vi "fill_tree.vi"(0 "Tree Refnum":refnum<vi>, 1 "Match String":string, 5 "Command Spec":T1, 7 "Operation":u16(ring) items=["Rebuild", "Add Items"], 9 "Property":string[](array[string]), 11 "Available Commands Pool":refnum<vi>, 12 "Group":string[](array[string]), 13 "Items to Insert":string[](array[string]), 14 "Sorting Method":u16) -> ()   [LabVIEW 2018]
uses:
  command_spec.ctl
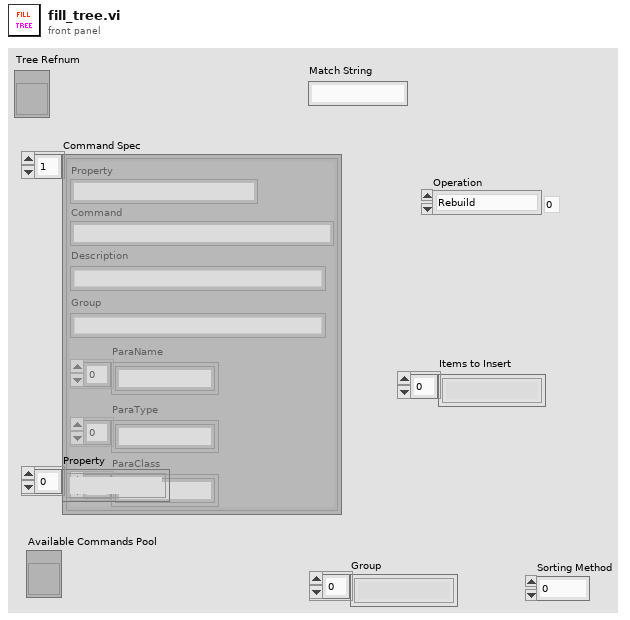
[diagram p1: front panel]
types:
  T1 = typedef "command_spec.ctl" = cluster{"Property":string, "Command":string, "Description":string, "Group":string, "ParaName":string[], "ParaType":string[], "ParaClass":string[]}[]
  T2 = cluster{"Left Cell String":string, "Child Text":string[], "Child Tag":string, "Item Indent":i32, "Child Only?":bool, "Glyph Index":i32}[]
  T3 = cluster{"Left Cell String":string, "Child Text":string[], "Child Tag":string, "Item Indent":i32, "Child Only?":bool, "Glyph Index":i32}
  T4 = cluster{"Property":string, "Command":string, "Description":string, "Group":string, "ParaName":string[], "ParaType":string[], "ParaClass":string[]}
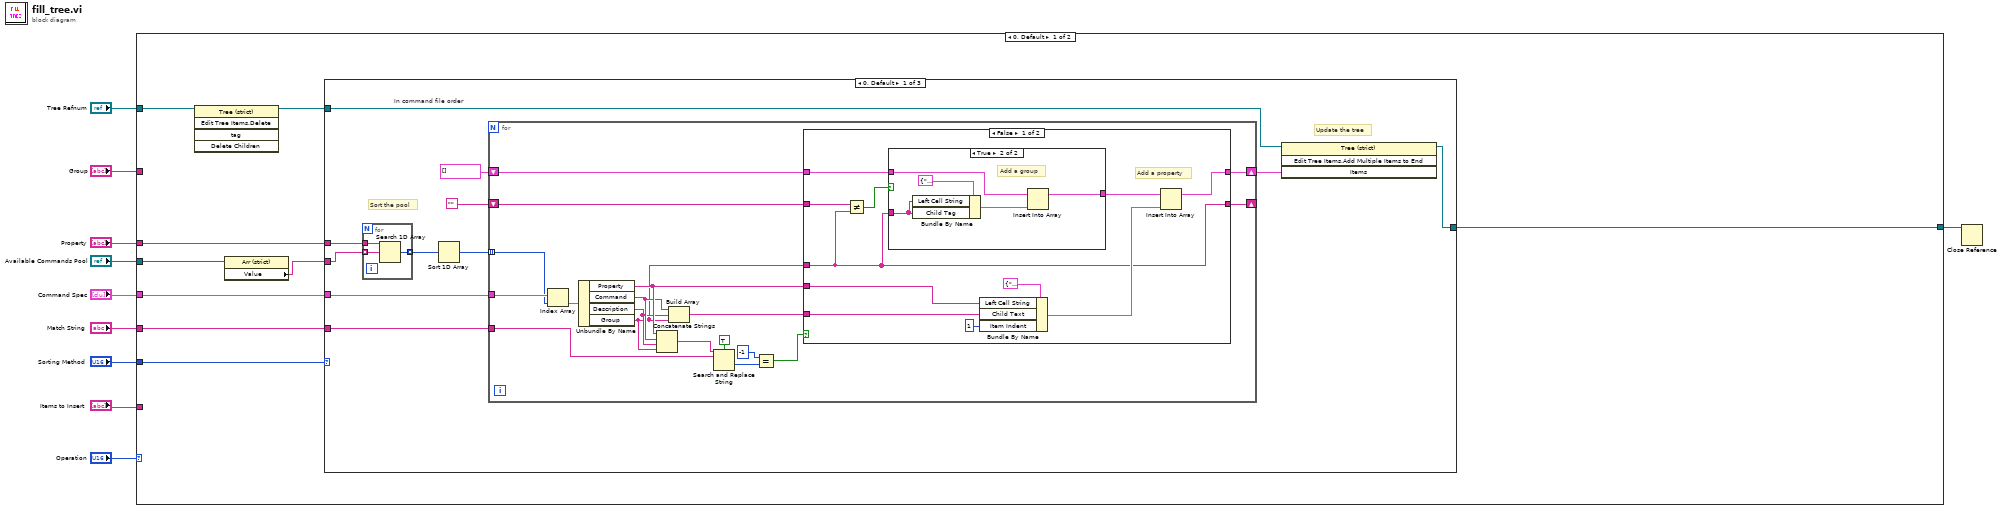
[diagram p0: block diagram]
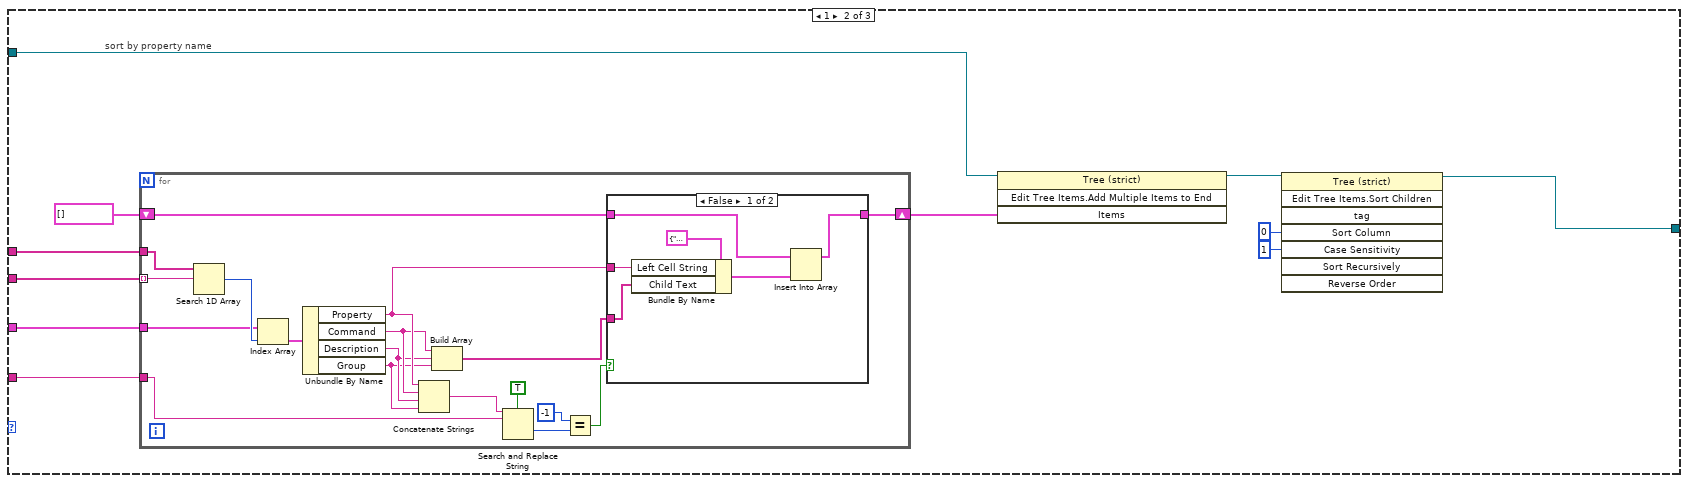
[diagram p4: hidden frame]
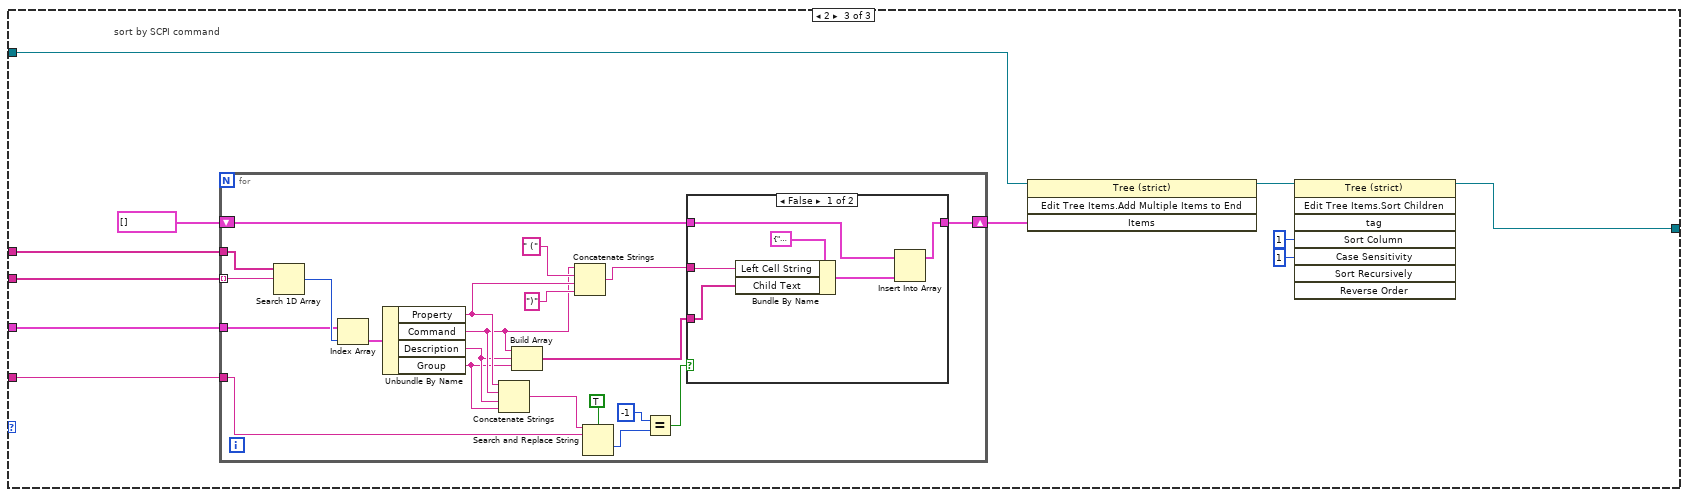
[diagram p6: hidden frame]
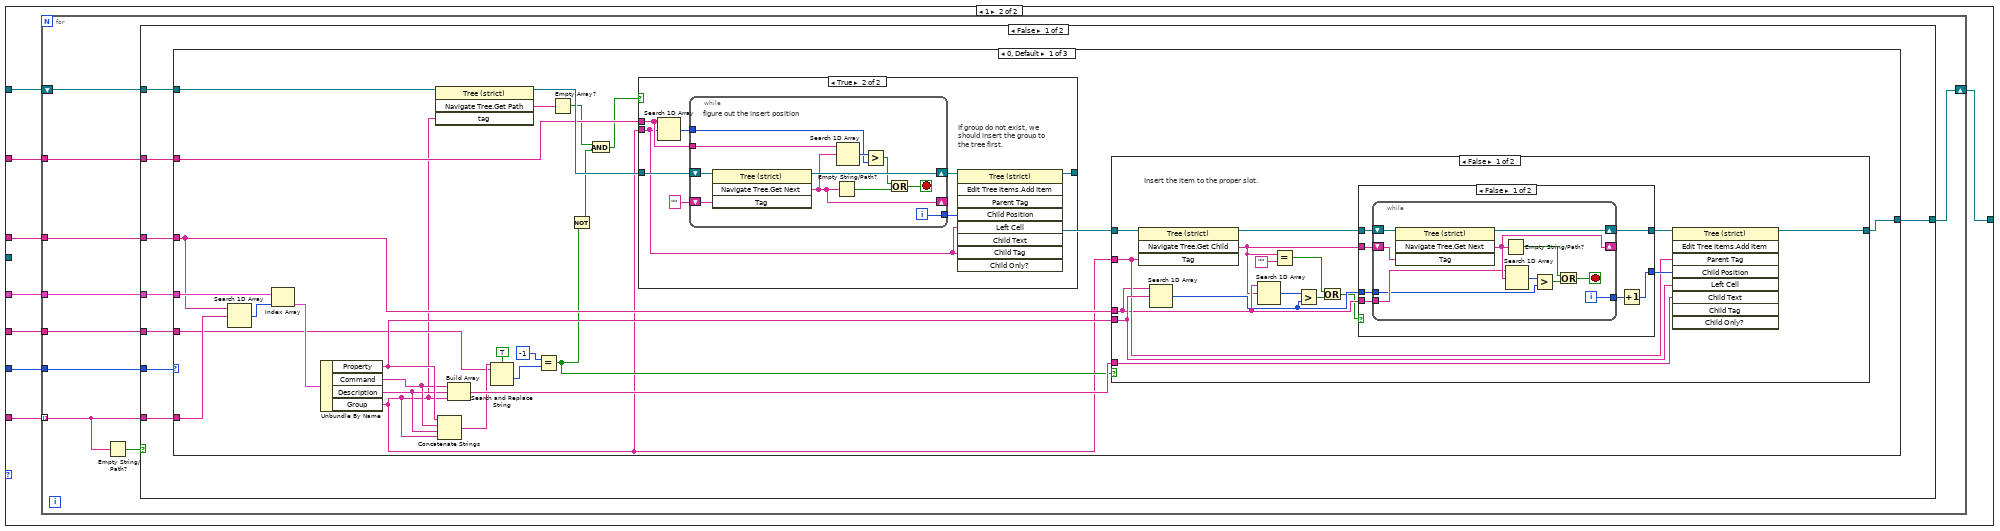
[diagram p8: hidden frame]
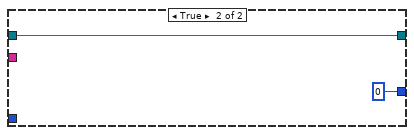
[diagram p9: hidden frame]
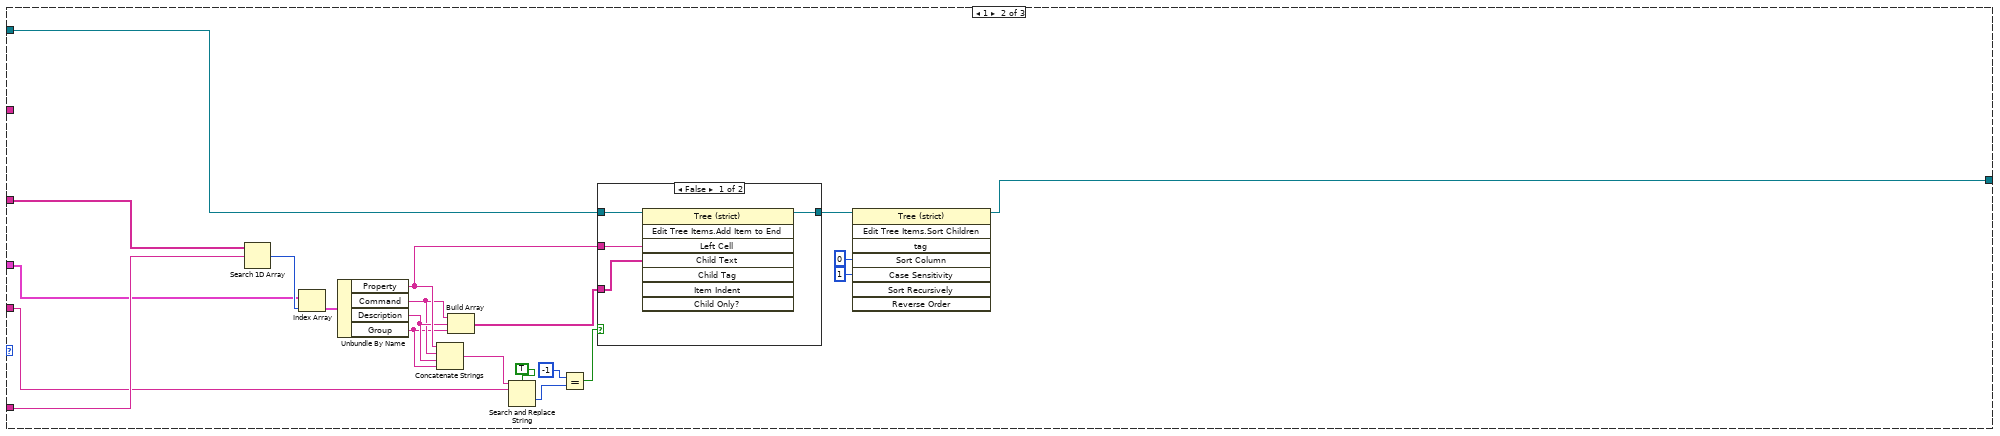
[diagram p12: hidden frame]
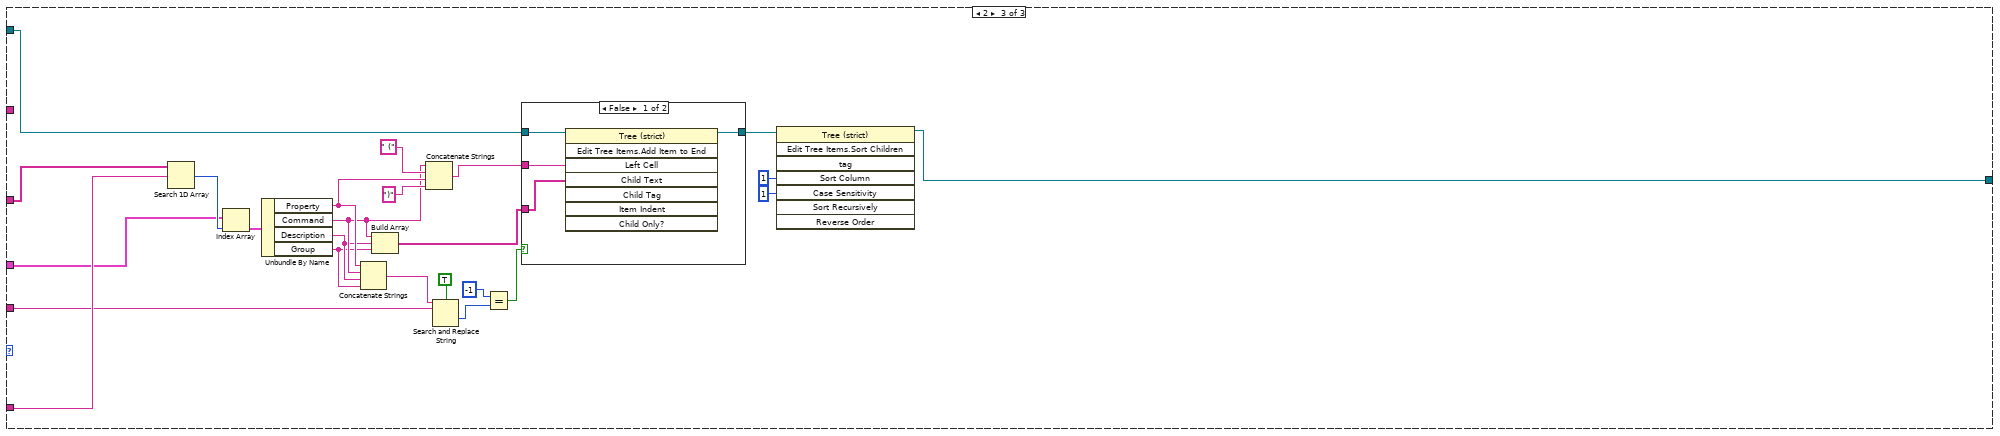
[diagram p14: hidden frame]
diagram:
  n1 = case shown="0, Default" "Operation" {
    tunnel: "Property" -> [w19 w152]
    tunnel: "Command Spec" -> [w18 w151]
    tunnel: [w17 w149] -> w8
    tunnel: "Sorting Method" -> [w16 w153]
    tunnel: "Match String" -> [w15 w150]
    tunnel: "Tree Refnum" -> [w13 w146]
    tunnel: "Available Commands Pool" -> [w12 _]
    tunnel: "Group" -> [_ w148]
    tunnel: "Items to Insert" -> [_ w147]
    frame 0, Default {
      n2 = invoke class="Tree (strict)" method="Edit Tree Items.Delete"(reference=w13) -> (reference out=w11:refnum<vi>)  [unwired: 4 in, 4 out]
      n3 = property class="Arr (strict)"(reference=w12) -> ("Value"=w14:string[])  [unwired: 1 in, 2 out]
      n4 = case shown="0, Default" w16 {
        tunnel: w19 -> [w23 w81 w117]
        tunnel: w14 -> [w22 w80 w116]
        tunnel: w18 -> [w28 w79 w115]
        tunnel: [w26 w75 w107] -> w17
        tunnel: w15 -> [w30 w78 w114]
        tunnel: w11 -> [w24 w72 w109]
        frame 0, Default {
          # "Sort the pool"
          # "Update the tree"
          # "In command file order"
          n5 = for {
            tunnel: w23 -> [w33]
            tunnel: w22 -> [w32] mode=indexing
            tunnel: [w31] -> w21 mode=indexing
            n6 = Search 1D Array(1D array=w33, element=w32) -> (index of element=w31:i32)  [unwired: 1 in]
          }
          n7 = Sort 1D Array(array=w21) -> (sorted array=w20:i32[])
          n8 = for {
            tunnel: w28 -> [w51]
            tunnel: w30 -> [w39]
            shift-right: [w44] -> _
            shift-left: "" -> [w43]
            shift-right: [w41] -> w27
            shift-left: T2 [] ("Property") -> [w42]
            tunnel: w20 -> [w34] mode=indexing
            n9 = Index Array(array=w51, index=w34) -> (element=w49:T4)
            n10 = Unbundle By Name(w49) -> ("Property"=w50:string, "Command"=w38:string, "Description"=w37:string, "Group"=w36:string)
            n11 = Concatenate Strings(w50, w38, w37, w36) -> (w45:string)
            n12 = Build Array(w38, w37, w36) -> (w35:string[])
            n13 = Search and Replace String(case sensitive?=TRUE ("ignore case? (F)"), input string=w45, search string=w39) -> (offset past replacement=w47:i32)  [unwired: 5 in, 3 out]
            n14 = Equal?(x=-1, y=w47) -> (x = y?=w40:bool)
            n15 = case shown="False" w40 {
              tunnel: w36 -> [w53 _]
              tunnel: w50 -> [w60 _]
              tunnel: [w53 w70] -> w44
              tunnel: w43 -> [w62 w70]
              tunnel: w42 -> [w57 w69]
              tunnel: [w54 w69] -> w41
              tunnel: w35 -> [w52 _]
              frame False {
                # "Add a property"
                n16 = Not Equal?(x=w62, y=w53) -> (x != y?=w55:bool)
                n17 = case shown="True" w55 {
                  tunnel: w53 -> [_ w68]
                  tunnel: w57 -> [w63 w65]
                  tunnel: [w63 w64] -> w56
                  frame False {
                  }
                  frame True {
                    # "Add a group"
                    n18 = Bundle By Name(cluster=T3 {"Left Cell String"="", "Child Text"=[], "Child Tag"="", "Item Indent"=0, "Child Only?"=FALSE, "Glyph Index"=0} ("element"), "Left Cell String"=w68, "Child Tag"=w68) -> (w66:T3)
                    n19 = Insert Into Array(array=w65, new element=w66) -> (w64:T2)  [unwired: 1 in]
                  }
                }
                n20 = Bundle By Name(cluster=T3 {"Left Cell String"="", "Child Text"=[], "Child Tag"="", "Item Indent"=0, "Child Only?"=FALSE, "Glyph Index"=0} ("element"), "Left Cell String"=w60, "Child Text"=w52, "Item Indent"=1) -> (w58:T3)
                n21 = Insert Into Array(array=w56, new element=w58) -> (w54:T2)  [unwired: 1 in]
              }
              frame True {
              }
            }
          }
          n22 = invoke class="Tree (strict)" method="Edit Tree Items.Add Multiple Items to End"(reference=w24, "Items"=w27) -> (reference out=w26:refnum<vi>)  [unwired: 2 in, 3 out]
        }
        frame 1 {
          # "sort by property name"
          n23 = for {
            tunnel: w80 -> [w98] mode=indexing
            tunnel: w81 -> [w99]
            tunnel: w79 -> [w96]
            tunnel: w78 -> [w91]
            shift-right: [w82] -> w73
            shift-left: T2 [] ("Property") -> [w83]
            n24 = Search 1D Array(1D array=w99, element=w98) -> (index of element=w97:i32)  [unwired: 1 in]
            n25 = Index Array(array=w96, index=w97) -> (element=w95:T4)
            n26 = Unbundle By Name(w95) -> ("Property"=w87:string, "Command"=w86:string, "Description"=w85:string, "Group"=w84:string)
            n27 = Concatenate Strings(w87, w86, w85, w84) -> (w90:string)
            n28 = Build Array(w86, w85, w84) -> (w88:string[])
            n29 = Search and Replace String(case sensitive?=TRUE ("ignore case? (F)"), input string=w90, search string=w91) -> (offset past replacement=w93:i32)  [unwired: 5 in, 3 out]
            n30 = Equal?(x=-1, y=w93) -> (x = y?=w89:bool)
            n31 = case shown="False" w89 {
              tunnel: w87 -> [w104 _]
              tunnel: w88 -> [w103 _]
              tunnel: w83 -> [w101 w106]
              tunnel: [w100 w106] -> w82
              frame False {
                n32 = Bundle By Name(cluster=T3 {"Left Cell String"="", "Child Text"=[], "Child Tag"="", "Item Indent"=0, "Child Only?"=FALSE, "Glyph Index"=0} ("element"), "Left Cell String"=w104, "Child Text"=w103) -> (w102:T3)
                n33 = Insert Into Array(array=w101, new element=w102) -> (w100:T2)  [unwired: 1 in]
              }
              frame True {
              }
            }
          }
          n34 = invoke class="Tree (strict)" method="Edit Tree Items.Add Multiple Items to End"(reference=w72, "Items"=w73) -> (reference out=w71:refnum<vi>)  [unwired: 2 in, 3 out]
          n35 = invoke class="Tree (strict)" method="Edit Tree Items.Sort Children"(reference=w71, "Sort Column"=0, "Case Sensitivity"=1) -> (reference out=w75:refnum<vi>)  [unwired: 5 in, 7 out]
        }
        frame 2 {
          # "sort by SCPI command"
          n36 = for {
            tunnel: w116 -> [w137] mode=indexing
            tunnel: w117 -> [w138]
            tunnel: w115 -> [w135]
            tunnel: w114 -> [w130]
            shift-right: [w118] -> w110
            shift-left: T2 [] ("Property") -> [w119]
            n37 = Search 1D Array(1D array=w138, element=w137) -> (index of element=w136:i32)  [unwired: 1 in]
            n38 = Index Array(array=w135, index=w136) -> (element=w134:T4)
            n39 = Unbundle By Name(w134) -> ("Property"=w123:string, "Command"=w122:string, "Description"=w121:string, "Group"=w120:string)
            n40 = Concatenate Strings(w123, w122, w121, w120) -> (w129:string)
            n41 = Build Array(w122, w121, w120) -> (w127:string[])
            n42 = Concatenate Strings(w122, " (" ("string"), w123, ")" ("string")) -> (w126:string)
            n43 = Search and Replace String(case sensitive?=TRUE ("ignore case? (F)"), input string=w129, search string=w130) -> (offset past replacement=w132:i32)  [unwired: 5 in, 3 out]
            n44 = Equal?(x=-1, y=w132) -> (x = y?=w128:bool)
            n45 = case shown="False" w128 {
              tunnel: w126 -> [w142 _]
              tunnel: w127 -> [w141 _]
              tunnel: w119 -> [w140 w145]
              tunnel: [w139 w145] -> w118
              frame False {
                n46 = Bundle By Name(cluster=T3 {"Left Cell String"="", "Child Text"=[], "Child Tag"="", "Item Indent"=0, "Child Only?"=FALSE, "Glyph Index"=0} ("element"), "Left Cell String"=w142, "Child Text"=w141) -> (w143:T3)
                n47 = Insert Into Array(array=w140, new element=w143) -> (w139:T2)  [unwired: 1 in]
              }
              frame True {
              }
            }
          }
          n48 = invoke class="Tree (strict)" method="Edit Tree Items.Add Multiple Items to End"(reference=w109, "Items"=w110) -> (reference out=w108:refnum<vi>)  [unwired: 2 in, 3 out]
          n49 = invoke class="Tree (strict)" method="Edit Tree Items.Sort Children"(reference=w108, "Sort Column"=1, "Case Sensitivity"=1) -> (reference out=w107:refnum<vi>)  [unwired: 5 in, 7 out]
        }
      }
    }
    frame 1 {
      n50 = for {
        tunnel: w153 -> [w162]
        tunnel: w152 -> [w161]
        tunnel: w151 -> [w160]
        tunnel: w150 -> [w159]
        tunnel: w148 -> [w156]
        tunnel: w147 -> [w155] mode=indexing
        shift-right: [w158] -> w149
        shift-left: w146 -> [w154]
        n51 = Empty String/Path?(string/path=w155) -> (empty?=w157:bool)
        n52 = case shown="False" w157 {
          tunnel: w162 -> [w170 _]
          tunnel: w154 -> [w169 w308]
          tunnel: w161 -> [w168 _]
          tunnel: w155 -> [w167 _]
          tunnel: w160 -> [w166 _]
          tunnel: w159 -> [w165 _]
          tunnel: [w164 w308] -> w158
          tunnel: w156 -> [w163 _]
          frame False {
            n53 = case shown="0, Default" w170 {
              tunnel: w167 -> [w194 w260 w286]
              tunnel: w169 -> [w195 w257 w283]
              tunnel: w168 -> [w180 w261 w287]
              tunnel: w166 -> [w181 w259 w285]
              tunnel: w165 -> [w182 w258 w284]
              tunnel: [w179 w256 w282] -> w164
              tunnel: w163 -> [w178 _ _]
              frame 0, Default {
                n54 = Search 1D Array(1D array=w180, element=w194) -> (index of element=w193:i32)  [unwired: 1 in]
                n55 = Index Array(array=w181, index=w193) -> (element=w189:T4)
                n56 = Unbundle By Name(w189) -> ("Property"=w187:string, "Command"=w173:string, "Description"=w172:string, "Group"=w171:string)
                n57 = invoke class="Tree (strict)" method="Navigate Tree.Get Path"(reference=w195, "tag"=w171) -> (reference out=w191:refnum<vi>, "Navigate Tree:Get Path"=w192:string[])  [unwired: 2 in, 2 out]
                n58 = Concatenate Strings(w187, w173, w172, w171) -> (w183:string)
                n59 = Build Array(w173, w172, w171) -> (w188:string[])
                n60 = Search and Replace String(case sensitive?=TRUE ("ignore case? (F)"), input string=w183, search string=w182) -> (offset past replacement=w185:i32)  [unwired: 5 in, 3 out]
                n61 = Equal?(x=-1, y=w185) -> (x = y?=w175:bool)
                n62 = Empty Array?(array=w192) -> (empty?=w177:bool)
                n63 = Not(x=w175) -> (.not. x?=w174:bool)
                n64 = And(x=w177, y=w174) -> (x .and. y?=w176:bool)
                n65 = case shown="True" w176 {
                  tunnel: w191 -> [w233 w240]
                  tunnel: w171 -> [_ w237]
                  tunnel: [w233 w241] -> w190
                  tunnel: w178 -> [_ w238]
                  frame False {
                  }
                  frame True {
                    # "If group do not exist, we should insert the group to the tree first."
                    n66 = Search 1D Array(1D array=w238, element=w237) -> (index of element=w236:i32)  [unwired: 1 in]
                    n67 = while {
                      tunnel: w238 -> [w250]
                      tunnel: w236 -> [w248]
                      tunnel: [w244] -> w235
                      shift-right: [w251] -> w239
                      shift-left: w240 -> [w252]
                      shift-right: [w242] -> _
                      shift-left: "" ("Tag") -> [w243]
                      i -> [w244]
                      stop <- w245 stop-if-true
                      # "figure out the insert position"
                      n68 = invoke class="Tree (strict)" method="Navigate Tree.Get Next"(reference=w252, "Tag"=w243) -> (reference out=w251:refnum<vi>, "Navigate Tree:Get Next Item"=w242:string)  [unwired: 2 in, 2 out]
                      n69 = Empty String/Path?(string/path=w242) -> (empty?=w247:bool)
                      n70 = Search 1D Array(1D array=w250, element=w242) -> (index of element=w249:i32)  [unwired: 1 in]
                      n71 = Greater?(x=w249, y=w248) -> (0:w246:bool)
                      n72 = Or(x=w246, y=w247) -> (x .or. y?=w245:bool)
                    }
                    n73 = invoke class="Tree (strict)" method="Edit Tree Items.Add Item"(reference=w239, "Child Position"=w235, "Left Cell"=w237, "Child Tag"=w237) -> (reference out=w241:refnum<vi>)  [unwired: 5 in, 8 out]
                  }
                }
                n74 = case shown="False" w175 {
                  tunnel: w190 -> [w208 w232]
                  tunnel: w188 -> [w211 _]
                  tunnel: w187 -> [w210 _]
                  tunnel: w171 -> [w204 _]
                  tunnel: [w196 w232] -> w179
                  tunnel: w180 -> [w203 _]
                  frame False {
                    # "Insert the item to the proper slot."
                    n75 = invoke class="Tree (strict)" method="Navigate Tree.Get Child"(reference=w208, "Tag"=w204) -> (reference out=w207:refnum<vi>, "Navigate Tree:Get Child"=w202:string)  [unwired: 2 in, 2 out]
                    n76 = Search 1D Array(1D array=w203, element=w210) -> (index of element=w200:i32)  [unwired: 1 in]
                    n77 = Search 1D Array(1D array=w203, element=w202) -> (index of element=w201:i32)  [unwired: 1 in]
                    n78 = Equal?(x=w202, y="") -> (x = y?=w199:bool)
                    n79 = Greater?(x=w201, y=w200) -> (0:w198:bool)
                    n80 = Or(x=w199, y=w198) -> (x .or. y?=w197:bool)
                    n81 = case shown="False" w197 {
                      tunnel: [w215 w231] -> w209
                      tunnel: w207 -> [w218 w231]
                      tunnel: [w212 0 ("Child Position")] -> w205
                      tunnel: w200 -> [w217 _]
                      tunnel: w203 -> [w216 _]
                      tunnel: w202 -> [w214 _]
                      frame False {
                        n82 = while {
                          shift-right: [w220] -> w215
                          shift-left: w218 -> [w229]
                          shift-right: [w227] -> _
                          shift-left: w214 -> [w228]
                          tunnel: w217 -> [w224]
                          tunnel: w216 -> [w226]
                          tunnel: [w219] -> w213
                          i -> [w219]
                          stop <- w221 stop-if-true
                          n83 = invoke class="Tree (strict)" method="Navigate Tree.Get Next"(reference=w229, "Tag"=w228) -> (reference out=w220:refnum<vi>, "Navigate Tree:Get Next Item"=w227:string)  [unwired: 2 in, 2 out]
                          n84 = Empty String/Path?(string/path=w227) -> (empty?=w223:bool)
                          n85 = Search 1D Array(1D array=w226, element=w227) -> (index of element=w225:i32)  [unwired: 1 in]
                          n86 = Greater?(x=w225, y=w224) -> (0:w222:bool)
                          n87 = Or(x=w223, y=w222) -> (x .or. y?=w221:bool)
                        }
                        n88 = Increment(x=w213) -> (x+1=w212:i32)
                      }
                      frame True {
                      }
                    }
                    n89 = invoke class="Tree (strict)" method="Edit Tree Items.Add Item"(reference=w209, "Parent Tag"=w204, "Child Position"=w205, "Left Cell"=w210, "Child Text"=w211) -> (reference out=w196:refnum<vi>)  [unwired: 4 in, 8 out]
                  }
                  frame True {
                  }
                }
              }
              frame 1 {
                n90 = Search 1D Array(1D array=w261, element=w260) -> (index of element=w273:i32)  [unwired: 1 in]
                n91 = Index Array(array=w259, index=w273) -> (element=w272:T4)
                n92 = Unbundle By Name(w272) -> ("Property"=w262:string, "Command"=w254:string, "Description"=w255:string, "Group"=w253:string)
                n93 = Concatenate Strings(w262, w254, w255, w253) -> (w268:string)
                n94 = Build Array(w254, w255, w253) -> (w266:string[])
                n95 = Search and Replace String(case sensitive?=TRUE ("ignore case? (F)"), input string=w268, search string=w258) -> (offset past replacement=w270:i32)  [unwired: 5 in, 3 out]
                n96 = Equal?(x=-1, y=w270) -> (x = y?=w267:bool)
                n97 = case shown="False" w267 {
                  tunnel: w257 -> [w277 w278]
                  tunnel: [w276 w278] -> w263
                  tunnel: w262 -> [w275 _]
                  tunnel: w266 -> [w274 _]
                  frame False {
                    n98 = invoke class="Tree (strict)" method="Edit Tree Items.Add Item to End"(reference=w277, "Left Cell"=w275, "Child Text"=w274) -> (reference out=w276:refnum<vi>)  [unwired: 5 in, 7 out]
                  }
                  frame True {
                  }
                }
                n99 = invoke class="Tree (strict)" method="Edit Tree Items.Sort Children"(reference=w263, "Sort Column"=0, "Case Sensitivity"=1) -> (reference out=w256:refnum<vi>)  [unwired: 5 in, 7 out]
              }
              frame 2 {
                n100 = Search 1D Array(1D array=w287, element=w286) -> (index of element=w302:i32)  [unwired: 1 in]
                n101 = Index Array(array=w285, index=w302) -> (element=w301:T4)
                n102 = Unbundle By Name(w301) -> ("Property"=w288:string, "Command"=w281:string, "Description"=w280:string, "Group"=w279:string)
                n103 = Concatenate Strings(w288, w281, w280, w279) -> (w297:string)
                n104 = Build Array(w281, w280, w279) -> (w295:string[])
                n105 = Concatenate Strings(w281, " (" ("string"), w288, ")" ("string")) -> (w291:string)
                n106 = Search and Replace String(case sensitive?=TRUE ("ignore case? (F)"), input string=w297, search string=w284) -> (offset past replacement=w299:i32)  [unwired: 5 in, 3 out]
                n107 = Equal?(x=-1, y=w299) -> (x = y?=w296:bool)
                n108 = case shown="False" w296 {
                  tunnel: w283 -> [w306 w307]
                  tunnel: [w305 w307] -> w292
                  tunnel: w291 -> [w304 _]
                  tunnel: w295 -> [w303 _]
                  frame False {
                    n109 = invoke class="Tree (strict)" method="Edit Tree Items.Add Item to End"(reference=w306, "Left Cell"=w304, "Child Text"=w303) -> (reference out=w305:refnum<vi>)  [unwired: 5 in, 7 out]
                  }
                  frame True {
                  }
                }
                n110 = invoke class="Tree (strict)" method="Edit Tree Items.Sort Children"(reference=w292, "Sort Column"=1, "Case Sensitivity"=1) -> (reference out=w282:refnum<vi>)  [unwired: 5 in, 7 out]
              }
            }
          }
          frame True {
          }
        }
      }
    }
  }
  n111 = Close Reference(reference=w8) -> ()  [unwired: 1 in, 1 out]
